vi "LM abx.vi"(0 "coefficients":dbl[](array[numeric]), 1 "model function":T2, 9 "output control":T1={"model function"=TRUE, "gradient"=TRUE}, 11 "error in (no error)":errorcluster, 12 "Y":dbl[](array[numeric]), 13 "X":dbl[](array[numeric]), 14 "Weight":dbl[](array[numeric])) -> (3 "number of function calls":i32, 4 "alpha":T4, 6 "beta":dbl[](array[numeric]), 8 "best fit":dbl[](array[numeric]), 10 "chiSqr":dbl, 15 "error out":errorcluster)   [LabVIEW 2014, in "NI_Gmath.lvlib"]
uses:
  NI_Gmath.lvlib
  RealMatrix.ctl
  LM model function.ctl
  LM model function reference.ctl
  LM_output select.ctl
  Real Outer Product.vi
  Array To Matrix - RA2.vi
  Add - RM,RM.vi
  NI_AALBase.lvlib
  NI_Matrix.lvlib
panel:
  # "Lev-Mar\nabx"
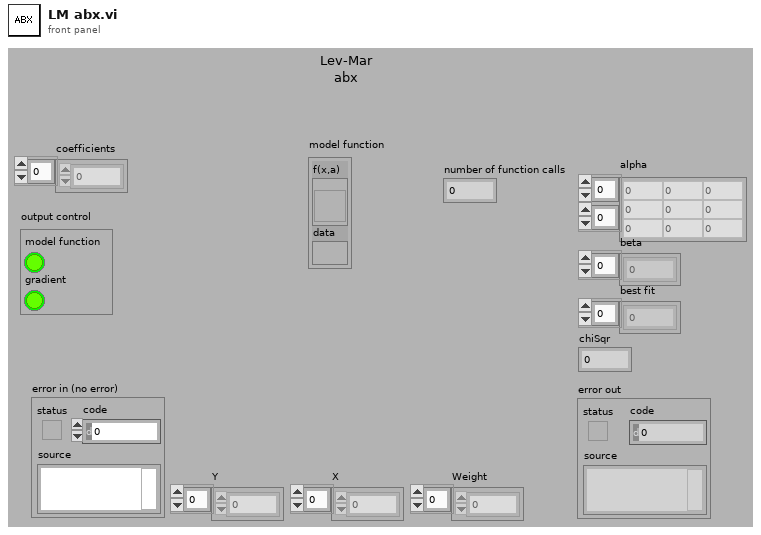
[diagram p1: front panel]
types:
  T1 = typedef "NI_Gmath.lvlib/LM_output select.ctl" = cluster{"model function":bool, "gradient":bool}
  T2 = typedef "NI_Gmath.lvlib/LM model function.ctl" = cluster{"f(x,a)":T3, "data":variant}
  T3 = typedef "NI_Gmath.lvlib/LM model function reference.ctl" = refnum<vi>
  T4 = typedef "NI_Matrix.lvlib/RealMatrix.ctl" = dbl[][]
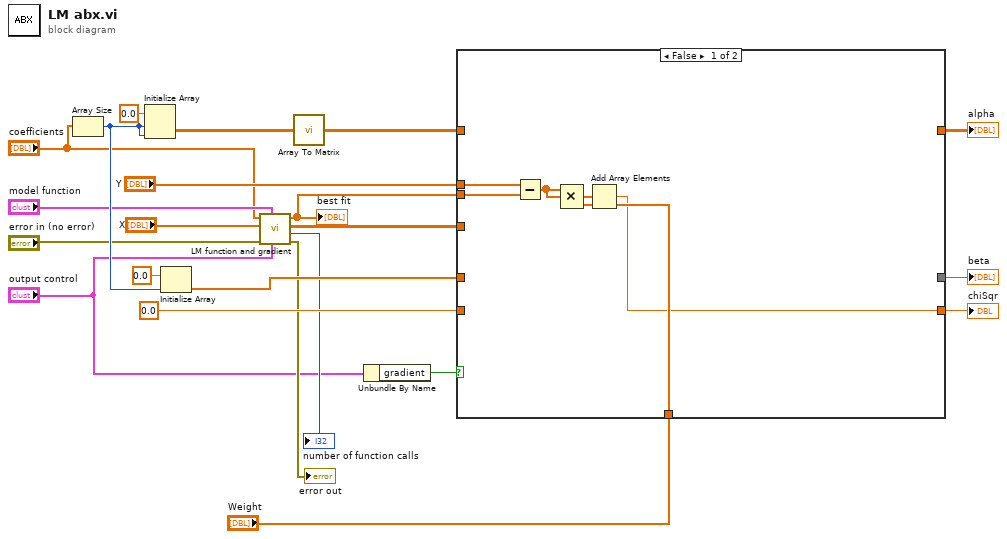
[diagram p0: block diagram]
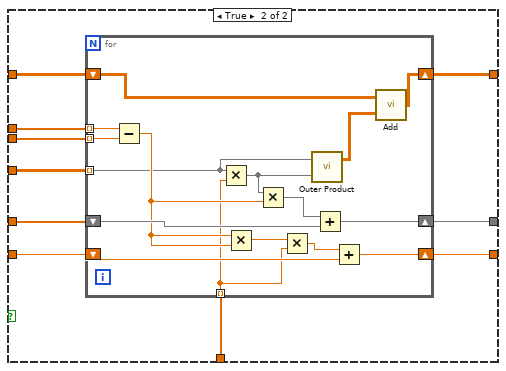
[diagram p2: hidden frame]
diagram:
  n1 = Array Size(array="coefficients") -> (size(s)=w22:i32)
  n2 = Initialize Array(0.0, w22, w22) -> (w19:dbl[][])
  n3 = Initialize Array(0.0, w22) -> (w20:dbl[])
  n4 = call "LM function and gradient.vi"("output control"="output control", "model function"="model function", "error in (no error)"="error in (no error)", "X"="X", "a"="coefficients") -> ("error out"=→"error out":errorcluster, "number of function calls"=→"number of function calls":i32, "gradient"=w7:dbl[][], "f(X)"=w8:dbl[])  [unwired: 3 in]
  "best fit" <- w8
  n5 = call-poly "Array To Matrix.vi"("Real 2D Array"=w19) -> ("Real Matrix"=w1:T4)
  n6 = Unbundle By Name("output control") -> ("gradient"=w3:bool)
  n7 = case shown="False" w3 {
    tunnel: w20 -> [_ w38]
    tunnel: w1 -> [_ w37]
    tunnel: [_ w29] -> w17
    tunnel: 0.0 -> [_ w36]
    tunnel: "Y" -> [w28 w31]
    tunnel: [_ w35] -> w14
    tunnel: [w23 w34] -> w13
    tunnel: w8 -> [w27 w30]
    tunnel: w7 -> [_ w32]
    tunnel: "Weight" -> [w25 w33]
    frame False {
      n8 = Subtract(x=w28, y=w27) -> (x-y=w26:dbl[])
      n9 = Compound Arithmetic op=MULTIPLY(w26, w26, w25) -> (w24:dbl[])
      n10 = Add Array Elements(numeric array=w24) -> (sum=w23:dbl)
    }
    frame True {
      n11 = for {
        shift-right: [w49] -> w29
        shift-left: w38 -> [w51]
        shift-right: [w39] -> w35
        shift-left: w37 -> [w41]
        shift-right: [w47] -> w34
        shift-left: w36 -> [w53]
        tunnel: w31 -> [w52] mode=indexing
        tunnel: w33 -> [w45] mode=indexing
        tunnel: w30 -> [w44] mode=indexing
        tunnel: w32 -> [w43] mode=indexing
        n12 = Subtract(x=w52, y=w44) -> (x-y=w48:dbl)
        n13 = Multiply(x=w43, y=w45) -> (x*y=w42:dbl[])
        n14 = Multiply(x=w48, y=w48) -> (x*y=w54:dbl)
        n15 = Multiply(x=w42, y=w48) -> (x*y=w50:dbl[])
        n16 = Multiply(x=w54, y=w45) -> (x*y=w46:dbl)
        n17 = call-poly "Outer Product.vi"("Y Vector"=w42, "X Vector"=w43) -> ("Outer Product"=w40:T4)  [unwired: 1 out]
        n18 = Add(x=w50, y=w51) -> (x+y=w49:dbl[])
        n19 = Add(x=w46, y=w53) -> (x+y=w47:dbl)
        n20 = call-poly "Add.vi"("Real Matrix B"=w40, "Real Matrix A"=w41) -> ("A + B"=w39:T4)
      }
    }
  }
  "alpha" <- w14
  "beta" <- w17
  "chiSqr" <- w13
